vi "Global 1.vi"() -> ()   [LabVIEW 2018]
panel:
  out "SequenceFilePath":string
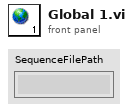
[diagram p1: front panel]
diagram:
